vi "linear_act_alpha.vi"() -> ()   [LabVIEW 2019]
uses:
  <vilib>/Instr/_visa.llb/VISA Configure Serial Port (Instr).vi
panel:
  in  "stop":bool
  in  "OK Button":bool
  out "String":string
  in  "Tab Control":enum32{"Move Stage", "Begin Experiment"}(tab)
  in  "-0.1mm":bool
  in  "+0.1mm":bool
  in  "-1mm":bool
  in  "+1mm":bool
  in  "-5mm":bool
  in  "+5mm Button":bool
  in  "- MOVE":bool
  in  "+ MOVE":bool
  in  "DIsplacement Depth (mm)":dbl
  in  "OK Button 2":bool
  in  "Frequency (Hz)":i16(knob) scale=0.0..7.0
  in  "VISA Resource Name":refnum<visa-resource-name>
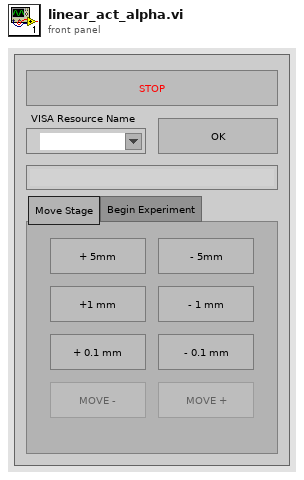
[diagram p1: front panel]
types:
  T1 = enum16{"Start", "Connect", "Idle", "Experiment", "Disconnect", "End", "Error"}
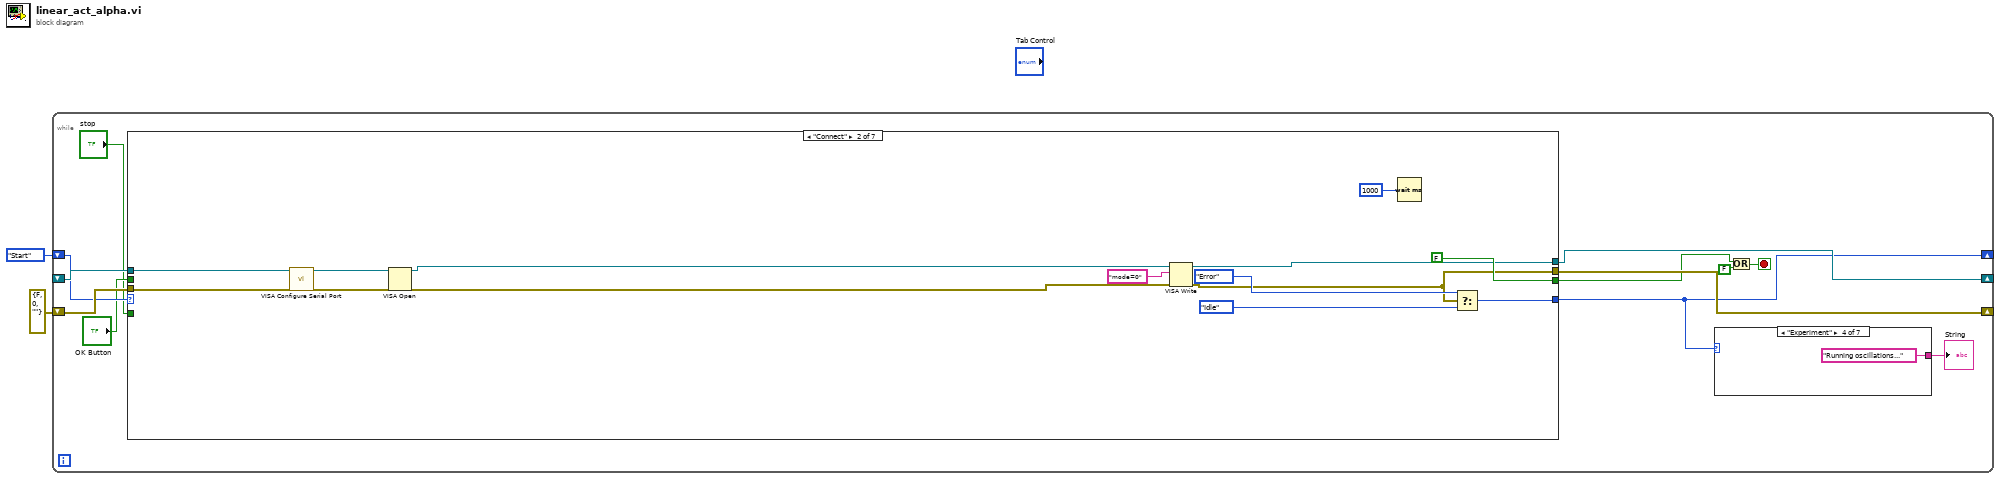
[diagram p0: block diagram]
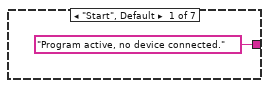
[diagram p2: hidden frame]
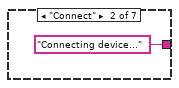
[diagram p3: hidden frame]
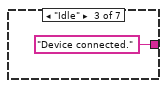
[diagram p4: hidden frame]
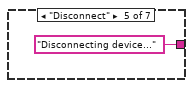
[diagram p5: hidden frame]
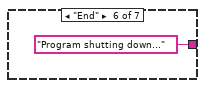
[diagram p6: hidden frame]
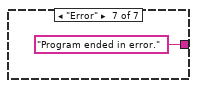
[diagram p7: hidden frame]
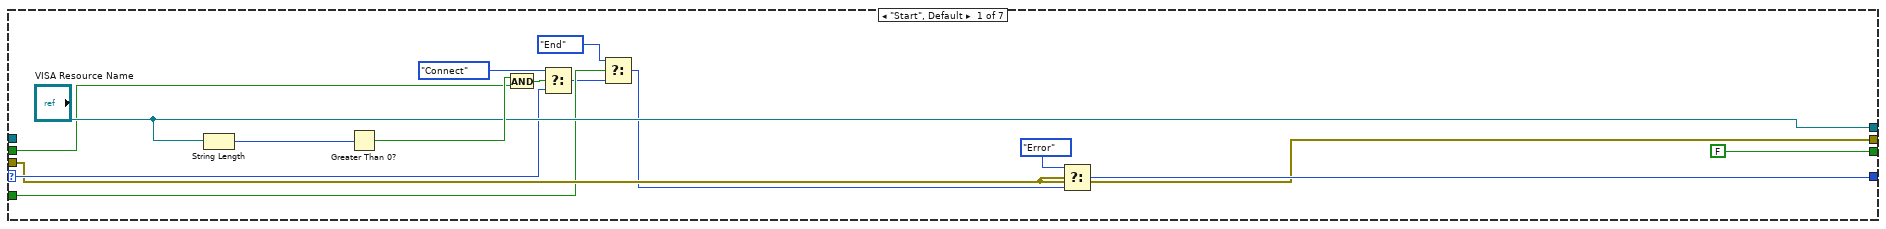
[diagram p8: hidden frame]
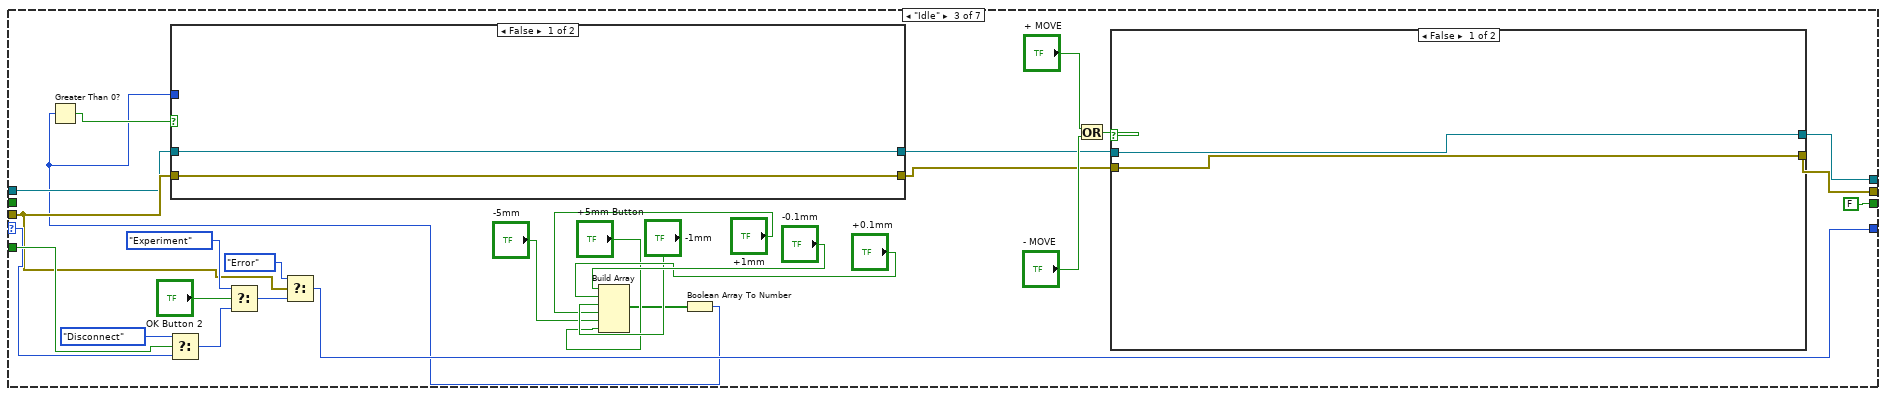
[diagram p9: hidden frame]
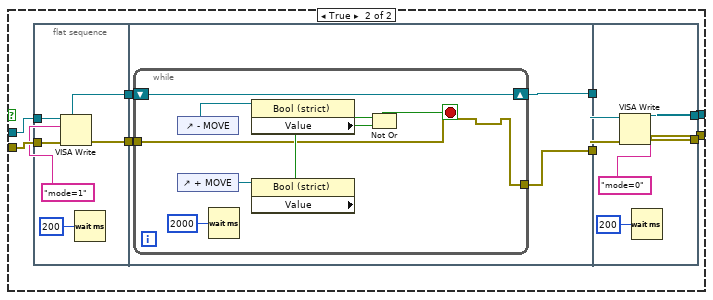
[diagram p10: hidden frame]
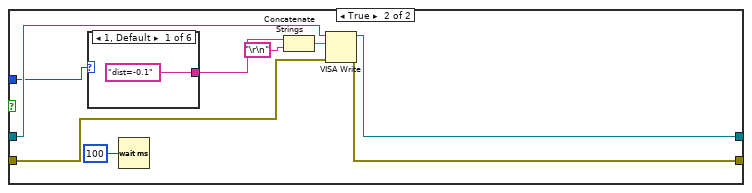
[diagram p11: hidden frame]
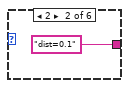
[diagram p12: hidden frame]
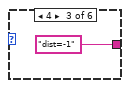
[diagram p13: hidden frame]
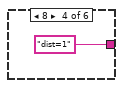
[diagram p14: hidden frame]
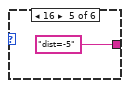
[diagram p15: hidden frame]
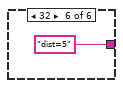
[diagram p16: hidden frame]
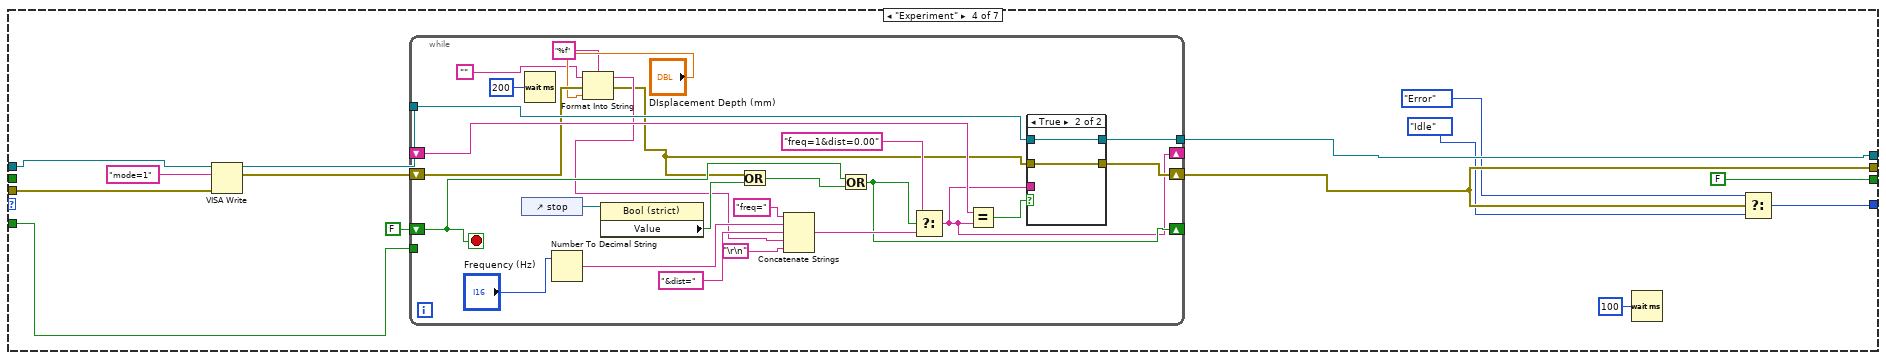
[diagram p17: hidden frame]
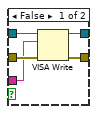
[diagram p18: hidden frame]
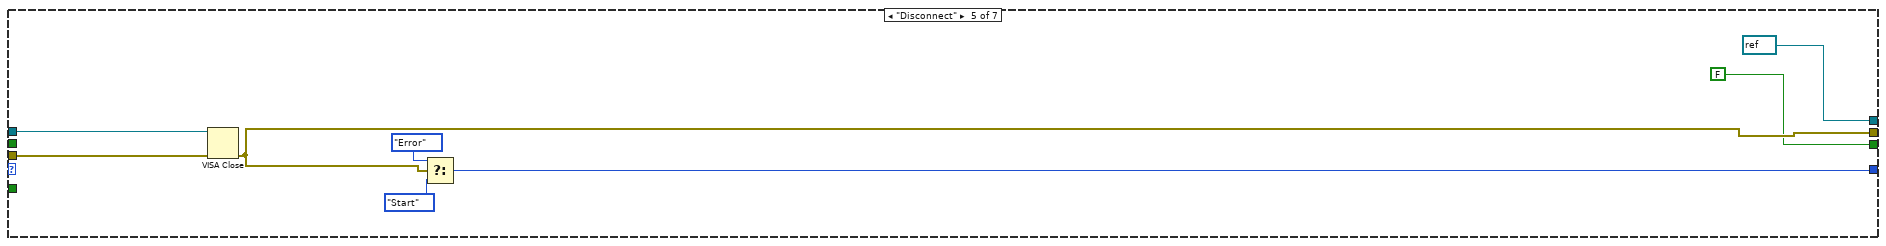
[diagram p19: hidden frame]
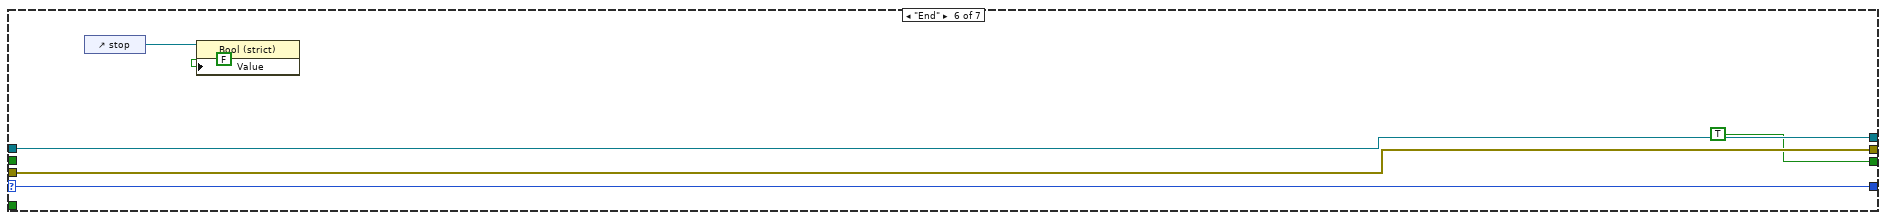
[diagram p20: hidden frame]
diagram:
  n1 = while {
    shift-right: [w6] -> _
    shift-left: T1."Start" -> [w12]
    shift-right: [w10] -> _
    shift-left: errorcluster {"status"=FALSE, "code"=0, "source"=""} ("error out") -> [w14]
    shift-right: [w11] -> _
    shift-left: _ -> [w13]
    stop <- w4 stop-if-true
    n2 = case shown="\"Connect\"" w12 {
      selector: w12 -> [w31 _ w76 _ _ w189 w195]
      tunnel: w14 -> [w27 w47 w68 w135 w182 w188 w192]
      tunnel: w13 -> [_ w48 w67 w134 w183 w187 w194]
      tunnel: [w30 w46 w69 w140 w180 w189 w195] -> w6
      tunnel: ["VISA Resource Name" w40 w63 w142 refnum<visa-resource-name> refnum ("VISA Resource Name") w187 w194] -> w11
      tunnel: [w27 w39 w62 w141 w181 w188 w192] -> w10
      tunnel: "stop" -> [w25 _ w78 w143 _ _ _]
      tunnel: "OK Button" -> [w33 _ _ _ _ _ _]
      tunnel: [FALSE FALSE FALSE FALSE FALSE TRUE TRUE] -> w3
      frame "Start", Default {
        n3 = String Length(string="VISA Resource Name") -> (length=w35:i32)
        n4 = Greater Than 0?(x=w35) -> (x > 0?=w36:bool)
        n5 = And(x=w36, y=w33) -> (x .and. y?=w32:bool)
        n6 = Select(t=T1."Connect", s=w32, f=w31) -> (s? t:f=w24:T1)
        n7 = Select(t=T1."End", s=w25, f=w24) -> (s? t:f=w26:T1)
        n8 = Select(t=T1."Error", s=w27, f=w26) -> (s? t:f=w30:T1)
      }
      frame "Connect" {
        n9 = call-poly "VISA Configure Serial Port"("VISA resource name"=w48, "error in (no error)"=w47) -> ("VISA resource name out"=w49:refnum<visa-resource-name>, "error out"=w50:errorcluster)  [unwired: 12 in]
        n10 = VISA Open(error in (no error)=w50, VISA resource name=w49) -> (VISA resource name=w42:refnum<visa-resource-name>, error out=w41:errorcluster)  [unwired: 3 in]
        n11 = VISA Write(VISA resource name=w42, write buffer="mode=0", error in (no error)=w41) -> (VISA resource name out=w40:refnum<visa-resource-name>, error out=w39:errorcluster)  [unwired: 1 out]
        n12 = Wait (ms)(milliseconds to wait=u32 1000) -> ()  [unwired: 1 out]
        n13 = Select(t=T1."Error", s=w39, f=T1."Idle") -> (s? t:f=w46:T1)
      }
      frame "Idle" {
        n14 = Select(t=T1."Disconnect", s=w78, f=w76) -> (s? t:f=w77:T1)
        n15 = Select(t=T1."Experiment", s="OK Button 2", f=w77) -> (s? t:f=w71:T1)
        n16 = Select(t=T1."Error", s=w68, f=w71) -> (s? t:f=w69:T1)
        n17 = Build Array("-0.1mm", "+0.1mm", "-1mm", "+1mm", "-5mm", "+5mm Button") -> (w51:bool[])
        n18 = Boolean Array To Number(Boolean array=w51) -> (number=w52:u32)
        n19 = Greater Than 0?(x=w52) -> (x > 0?=w53:bool)
        n20 = case shown="False" w53 {
          tunnel: w68 -> [w114 w123]
          tunnel: [w114 w122] -> w54
          tunnel: w67 -> [w113 w117]
          tunnel: [w113 w121] -> w55
          tunnel: w52 -> [_ w116]
          frame False {
          }
          frame True {
            n21 = case shown="1, Default" w116 {
              tunnel: ["dist=-0.1" ("write buffer") "dist=0.1" ("write buffer") "dist=-1" ("write buffer") "dist=1" ("write buffer") "dist=-5" ("write buffer") "dist=5" ("write buffer")] -> w115
              frame 1, Default {
              }
              frame 2 {
              }
              frame 4 {
              }
              frame 8 {
              }
              frame 16 {
              }
              frame 32 {
              }
            }
            n22 = Wait (ms)(milliseconds to wait=u32 100) -> ()  [unwired: 1 out]
            n23 = Concatenate Strings(w115, "\r\n") -> (w119:string)
            n24 = VISA Write(VISA resource name=w117, write buffer=w119, error in (no error)=w123) -> (VISA resource name out=w121:refnum<visa-resource-name>, error out=w122:errorcluster)  [unwired: 1 out]
          }
        }
        n25 = Or(x="+ MOVE", y="- MOVE") -> (x .or. y?=w65:bool)
        n26 = case shown="False" w65 {
          tunnel: w55 -> [w80 w86]
          tunnel: [w80 w82] -> w63
          tunnel: w54 -> [w79 w87]
          tunnel: [w79 w83] -> w62
          frame False {
          }
          frame True {
            n27 = flat-sequence {
              tunnel: [w92] -> w88
              tunnel: w87 -> [w94]
              tunnel: w86 -> [w93]
              tunnel: [w90] -> w81
              tunnel: w88 -> [w96]
              tunnel: [w98] -> w85
              tunnel: [w97] -> w84
              tunnel: w81 -> [w95]
              tunnel: w85 -> [w111]
              tunnel: w84 -> [w112]
              tunnel: [w110] -> w83
              tunnel: [w109] -> w82
              frame #0 {
                n28 = VISA Write(VISA resource name=w93, write buffer="mode=1", error in (no error)=w94) -> (VISA resource name out=w90:refnum<visa-resource-name>, error out=w92:errorcluster)  [unwired: 1 out]
                n29 = Wait (ms)(milliseconds to wait=u32 200) -> ()  [unwired: 1 out]
              }
              frame #1 {
                n30 = while {
                  shift-right: [w100] -> w98
                  shift-left: w95 -> [w100]
                  tunnel: [w99] -> w97
                  tunnel: w96 -> [w99]
                  stop <- w102 stop-if-true
                  n31 = control-ref of="- MOVE"() -> (w105:refnum<vi>)
                  n32 = control-ref of="+ MOVE"() -> (w106:refnum<vi>)
                  n33 = Wait (ms)(milliseconds to wait=u32 2000) -> ()  [unwired: 1 out]
                  n34 = property on="Property Node" class="Bool (strict)"(reference=w105) -> ("Value"=w103:bool)  [unwired: 1 in, 2 out]
                  n35 = property on="Property Node" class="Bool (strict)"(reference=w106) -> ("Value"=w104:bool)  [unwired: 1 in, 2 out]
                  n36 = Not Or(1:w103, 2:w104) -> (0:w102:bool)
                }
              }
              frame #2 {
                n37 = VISA Write(VISA resource name=w111, write buffer="mode=0", error in (no error)=w112) -> (VISA resource name out=w109:refnum<visa-resource-name>, error out=w110:errorcluster)  [unwired: 1 out]
                n38 = Wait (ms)(milliseconds to wait=u32 200) -> ()  [unwired: 1 out]
              }
            }
          }
        }
      }
      frame "Experiment" {
        n39 = VISA Write(VISA resource name=w134, write buffer="mode=1", error in (no error)=w135) -> (VISA resource name out=w133:refnum<visa-resource-name>, error out=w136:errorcluster)  [unwired: 1 out]
        n40 = while {
          tunnel: [w162] -> w142
          shift-right: [w163] -> w141
          shift-left: w136 -> [w147]
          tunnel: w133 -> [w160]
          shift-right: [w155] -> _
          shift-left: FALSE -> [w157]
          tunnel: w143 -> [_]
          shift-right: [w152] -> _
          shift-left: _ -> [w153]
          stop <- w157 stop-if-true
          n41 = control-ref of="stop"() -> (w151:refnum<vi>)
          n42 = Wait (ms)(milliseconds to wait=u32 200) -> ()  [unwired: 1 out]
          n43 = Number To Decimal String(number="Frequency (Hz)") -> (decimal integer string=w166:string)  [unwired: 1 in]
          n44 = Format Into String(format string="%f", initial string="", error in=w147, "DIsplacement Depth (mm)") -> (resulting string=w149:string, error out=w148:errorcluster)
          n45 = property on="Property Node" class="Bool (strict)"(reference=w151) -> ("Value"=w150:bool)  [unwired: 1 in, 2 out]
          n46 = Or(x=w148, y=w150) -> (x .or. y?=w156:bool)
          n47 = Concatenate Strings("freq=", w166, "&dist=", w149, "\r\n") -> (w159:string)
          n48 = Or(x=w157, y=w156) -> (x .or. y?=w155:bool)
          n49 = Select(t="freq=1&dist=0.00", s=w155, f=w159) -> (s? t:f=w152:string)
          n50 = Equal?(x=w153, y=w152) -> (x = y?=w154:bool)
          n51 = case shown="True" w154 {
            tunnel: [w173 w174] -> w163
            tunnel: [w172 w175] -> w162
            tunnel: w160 -> [w171 w175]
            tunnel: w148 -> [w170 w174]
            tunnel: w152 -> [w169 _]
            frame False {
              n52 = VISA Write(VISA resource name=w171, write buffer=w169, error in (no error)=w170) -> (VISA resource name out=w172:refnum<visa-resource-name>, error out=w173:errorcluster)  [unwired: 1 out]
            }
            frame True {
            }
          }
        }
        n53 = Wait (ms)(milliseconds to wait=u32 100) -> ()  [unwired: 1 out]
        n54 = Select(t=T1."Error", s=w141, f=T1."Idle") -> (s? t:f=w140:T1)
      }
      frame "Disconnect" {
        n55 = VISA Close(VISA resource name=w183, error in (no error)=w182) -> (error out=w181:errorcluster)
        n56 = Select(t=T1."Error", s=w181, f=T1."Start") -> (s? t:f=w180:T1)
      }
      frame "End" {
        n57 = control-ref of="stop"() -> (w184:refnum<vi>)
        n58 = property on="Property Node" class="Bool (strict)"(reference=w184, "Value"=FALSE ("stop")) -> ()  [unwired: 1 in, 2 out]
      }
      frame "Error" {
        n59 = call <vilib>:"Simple Error Handler.vi"("error in (no error)"=w192) -> ()  [unwired: 4 in, 5 out]
        n60 = control-ref of="stop"() -> (w190:refnum<vi>)
        n61 = property on="Property Node" class="Bool (strict)"(reference=w190, "Value"=FALSE ("stop")) -> ()  [unwired: 1 in, 2 out]
      }
    }
    n62 = case shown="\"Experiment\"" w6 {
      tunnel: ["Program active, no device connected." "Connecting device..." "Device connected." "Running oscillations..." "Disconnecting device..." "Program shutting down..." "Program ended in error."] -> w7
      frame "Start", Default {
      }
      frame "Connect" {
      }
      frame "Idle" {
      }
      frame "Experiment" {
      }
      frame "Disconnect" {
      }
      frame "End" {
      }
      frame "Error" {
      }
    }
    "String" <- w7
    n63 = Or(x=w3, y=FALSE) -> (x .or. y?=w4:bool)
  }
